vi "Close Semaphore.vi"(8 "error in (no error)":errorcluster caption="entrée d'erreur (pas d'erreur)", 11 "Class Instrument (Default) en entrée":refnum<class "Class Instrument (Default).lvclass">) -> (0 "error out":errorcluster caption="sortie d'erreur", 3 "Class Instrument (Default) en sortie":refnum<class "Class Instrument (Default).lvclass">)   [LabVIEW 2020, in "Library Instrument & Equipement.lvlib" / "Library Instruments.lvlib" / "Class Instrument (Default).lvclass"]
uses:
  Class Instrument (Default).lvclass
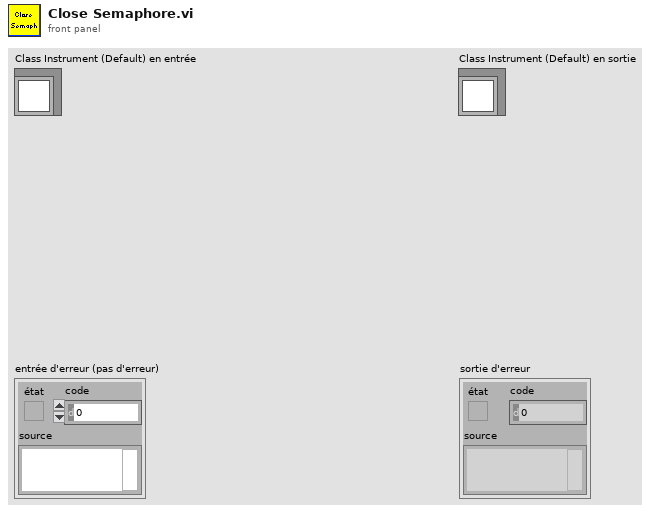
[diagram p1: front panel]
types:
  T1 = typedef "Semaphore RefNum" = refnum<k1>
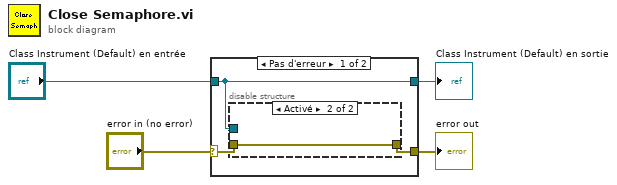
[diagram p0: block diagram]
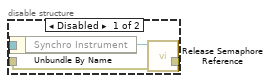
[diagram p2: hidden frame]
diagram:
  n1 = case shown="Pas d'erreur" "error in (no error)" {
    selector: "error in (no error)" -> [w6 w14]
    tunnel: [w5 w14] -> w3
    tunnel: [w7 w13] -> w1
    tunnel: "Class Instrument (Default) en entrée" -> [w7 w13]
    frame No Error {
      n2 = disable-structure shown="Activé" {
        disable-tunnel: w7 -> [w10 _]
        disable-tunnel: w6 -> [w9 w12]
        disable-tunnel: [w8 w12] -> w5
        frame Disabled {
          n3 = Unbundle By Name(w10) -> ("Synchro Instrument"=w11:T1)
          n4 = call <vilib>:"Release Semaphore Reference.vi"("error in (no error)"=w9, "semaphore"=w11) -> ("error out"=w8:errorcluster)  [unwired: 8 in, 1 out]
        }
        frame Enabled {
        }
      }
    }
    frame Error {
    }
  }
  "error out" <- w3
  "Class Instrument (Default) en sortie" <- w1
